vi "FlattenTOAPsetup.vi"() -> ()   [LabVIEW 2015]
panel:
  out "xml string":string
  in  "Cluster":T1={"textOrigin"={"x"=0, "y"=0}, "desired font(Application)"=enum."System Font", "[user-specified font]"={"Font Name:"="", "Size"=0, "Strikeout?"=FALSE, "Italic?"=FALSE, "Underline?"=FALSE, "Outline?"=FALSE, "Shadow?"=FALSE, "Bold?"=FALSE}}
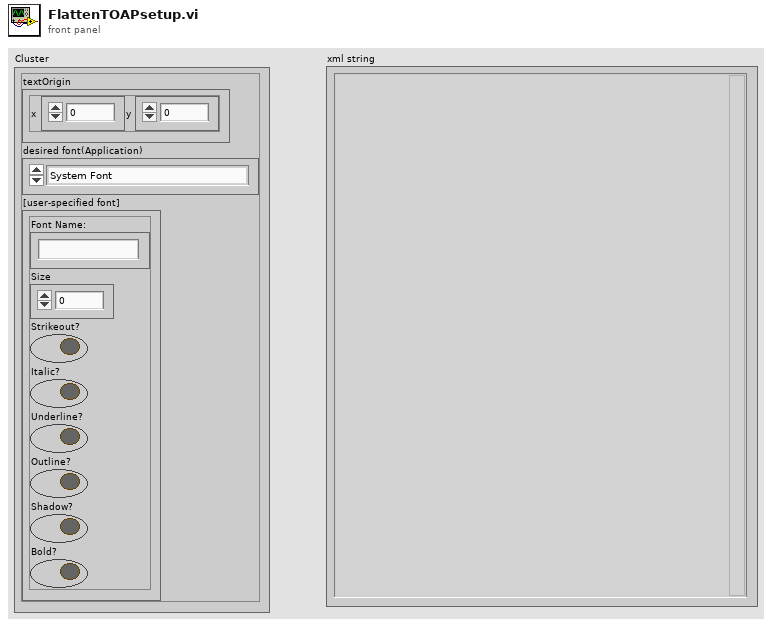
[diagram p1: front panel]
types:
  T1 = cluster{"textOrigin":cluster{"x":i16, "y":i16}, "desired font(Application)":enum16{"User-specified Font", "Application Font", "System Font", "Dialog Font"}, "[user-specified font]":cluster{"Font Name:":string, "Size":i16, "Strikeout?":bool, "Italic?":bool, "Underline?":bool, "Outline?":bool, "Shadow?":bool, "Bold?":bool}}
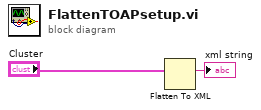
[diagram p0: block diagram]
diagram:
  n1 = Flatten To XML(anything="Cluster") -> (xml string=→"xml string":string)
